vi "Save AVI as PNGs.vi"() -> ()   [LabVIEW 2013]
panel:
  out "error out":errorcluster
  in  "error in (no error)":errorcluster
  in  "Destination Directory":path
  in  "AVI Path":path
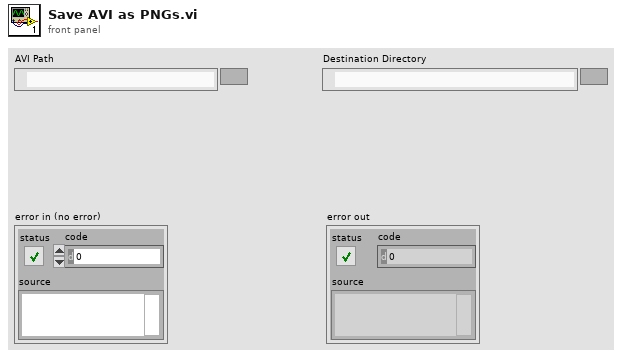
[diagram p1: front panel]
types:
  T1 = typedef "IMAQ Image.ctl" = refnum<image>
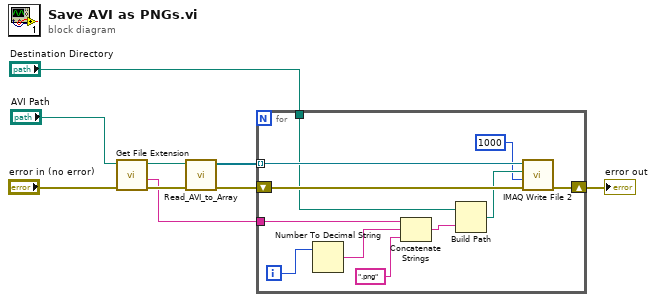
[diagram p0: block diagram]
diagram:
  n1 = call <vilib>:"Get File Extension.vi"("error in (no error)"="error in (no error)", "file"="AVI Path") -> ("error out"=w5:errorcluster, "filename without extension"=w3:string, "dup file"=w4:path)  [unwired: 6 in, 1 out]
  n2 = call "Read_AVI_to_Array.vi"("Error in (no error)"=w5, "AVI Path"=w4) -> ("Error out"=w8:errorcluster, "Image Array"=w9:T1[])  [unwired: 7 in, 1 out]
  n3 = for {
    tunnel: w9 -> [w17] mode=indexing
    shift-right: [w19] -> w1
    shift-left: w8 -> [w18]
    tunnel: "Destination Directory" -> [w10]
    tunnel: w3 -> [w12]
    i -> [w20]
    n4 = Number To Decimal String(number=w20) -> (decimal integer string=w14:string)  [unwired: 1 in]
    n5 = Concatenate Strings(w12, w14, ".png" ("string")) -> (w11:string)
    n6 = Build Path(base path=w10, name or relative path=w11) -> (appended path=w16:path)
    n7 = call-poly "IMAQ Write File 2"("error in (no error)"=w18, "Image Quality"=u32 1000, "File Path"=w16, "Image"=w17) -> ("error out"=w19:errorcluster)  [unwired: 6 in, 1 out]
  }
  "error out" <- w1
